vi "MotionControl.vi"(7 "Control Time":i32=500, 8 "error in":errorcluster, 9 "Samples":i32=10, 10 "InputSpeed":dbl, 11 "MotorControlDevRef":T1={"DeviceStatus"={"status"=FALSE, "code"=0, "source"=""}, "Type"=enum."PWM", "PWM"={"Controller"=enum."Controller 1", "PWM Channel"=enum."Invalid", "DeadBand"={"Name"="", "maxPositivePwm"=0, "minPositivePwm"=0, "centerPwm"=0, "maxNegativePwm"=0, "minNegativePwm"=0, "angularRange"=0}}, "CAN"={"Device Number"=0, "Control Mode"=enum."Percent VBus", "Semaphore"=refnum, "Max Vout"=12.0, "TalonSRX Control Mode"=enum."Percent VBus"}, "Invert"=FALSE, "TransformRef"=refnum, "InvTransformRef"=refnum}) -> ()   [LabVIEW 2014]
uses:
  <vilib>/Rock Robotics/WPI/MotorControl/WPI_MotorControlDeviceRef.ctl
  <vilib>/Rock Robotics/WPI/MotorControl/WPI_MotorControlType.ctl
  <vilib>/Rock Robotics/SystemInterfaces/Typedef/FPGA_TypedefDigitalModule.ctl
  <vilib>/Rock Robotics/SystemInterfaces/DIO/FPGA_DIOPWMChannel.ctl
  <vilib>/Rock Robotics/WPI/PWM/WPI_PWMDeadband.ctl
  <vilib>/Rock Robotics/WPI/CAN/Jaguar/SubVIs/WPI_CANJaguar_ControlMode.ctl
  <vilib>/Rock Robotics/WPI/CAN/TalonSRX/WPI_CANTalonSRX_APIControlMode.ctl
  <vilib>/Rock Robotics/WPI/PWM/WPI_PWMTransform_ConPane.ctl
panel:
  out "Waveform Chart":dbl(graph)
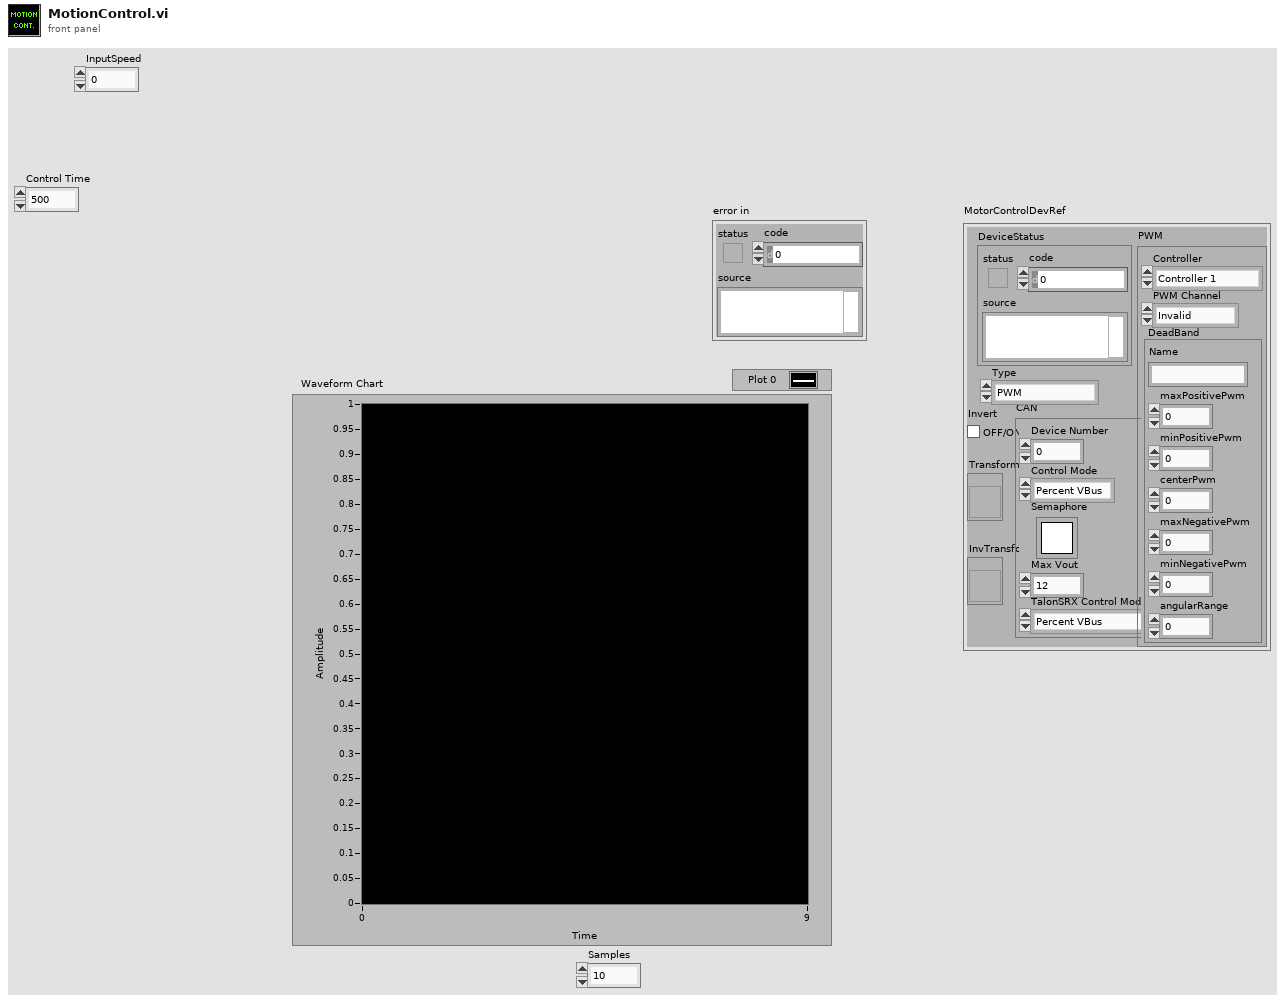
[diagram p1: front panel]
types:
  T1 = typedef "WPI_MotorControlDeviceRef.ctl" = cluster{"DeviceStatus":errorcluster, "Type":T2, "PWM":cluster{"Controller":T3, "PWM Channel":T4, "DeadBand":T5}, "CAN":cluster{"Device Number":u8, "Control Mode":T6, "Semaphore":T7, "Max Vout":dbl, "TalonSRX Control Mode":T8}, "Invert":bool, "TransformRef":T9, "InvTransformRef":T9}
  T2 = typedef "WPI_MotorControlType.ctl" = enum16{"PWM", "CAN", "CANTalonSRX"}
  T3 = typedef "FPGA_TypedefDigitalModule.ctl" = enum16{"Controller 1"}
  T4 = typedef "FPGA_DIOPWMChannel.ctl" = enum8{"PWM 0", "PWM 1", "PWM 2", "PWM 3", "PWM 4", "PWM 5", "PWM 6", "PWM 7", "PWM 8", "PWM 9", "PWM MXP 0", "PWM MXP 1", "PWM MXP 2", "PWM MXP 3", "PWM MXP 4", "PWM MXP 5", "PWM MXP 6", "PWM MXP 7", "PWM MXP 8", "PWM MXP 9", "Invalid"}
  T5 = typedef "WPI_PWMDeadband.ctl" = cluster{"Name":string, "maxPositivePwm":i32, "minPositivePwm":i32, "centerPwm":i32, "maxNegativePwm":i32, "minNegativePwm":i32, "angularRange":u16}
  T6 = typedef "WPI_CANJaguar_ControlMode.ctl" = enum8{"Percent VBus", "Current", "Speed", "Position", "Voltage"}
  T7 = typedef "Semaphore RefNum" = refnum<k1>
  T8 = typedef "WPI_CANTalonSRX_APIControlMode.ctl" = enum8{"Percent VBus", "Speed", "Position", "Slave", "Unchanged / Invalid"}
  T9 = typedef "WPI_PWMTransform_ConPane.ctl" = refnum<vi>
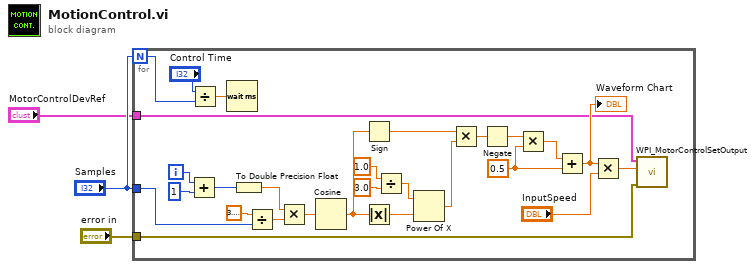
[diagram p0: block diagram]
diagram:
  n1 = for {
    N: "Samples" -> [w6]
    tunnel: "MotorControlDevRef" -> [w13]
    tunnel: "error in" -> [w12]
    tunnel: "Samples" -> [w9]
    i -> [w30]
    w19 = 0.5 ("y")
    n2 = Add(x=w30, y=1) -> (x+y=w11:i32)
    n3 = Divide(x="Control Time", y=w6) -> (x/y=w5:dbl)
    n4 = Wait (ms)(milliseconds to wait=w5) -> ()  [unwired: 1 out]
    n5 = To Double Precision Float(number=w11) -> (double precision float=w26:dbl)
    n6 = Divide(x=3.141592653589793, y=w9) -> (x/y=w27:dbl)
    n7 = Multiply(x=w26, y=w27) -> (x*y=w28:dbl)
    n8 = Cosine(x=w28) -> (cos(x)=w17:dbl)
    n9 = Sign(1:w17) -> (0:w15:dbl)
    n10 = Absolute Value(x=w17) -> (abs(x)=w18:dbl)
    n11 = Divide(x=1.0, y=3.0) -> (x/y=w25:dbl)
    n12 = Power Of X(1:w18, 2:w25) -> (0:w22:dbl)
    n13 = Multiply(x=w15, y=w22) -> (x*y=w16:dbl)
    n14 = Negate(x=w16) -> (-x=w21:dbl)
    n15 = Multiply(x=w21, y=w19) -> (x*y=w20:dbl)
    n16 = Add(x=w20, y=w19) -> (x+y=w14:dbl)
    "Waveform Chart" <- w14
    n17 = Multiply(x=w14, y="InputSpeed") -> (x*y=w7:dbl)
    n18 = call <vilib>:"WPI_MotorControlSetOutput.vi"("error in (no error)"=w12, "Output"=w7, "MotorControlDevRef"=w13) -> ()  [unwired: 6 in, 3 out]
  }
